vi "write key.vi"(8 "error in (no error)":errorcluster, 10 "key":u8, 11 "uri":string) -> (0 "error out":errorcluster, 2 "key out":u8, 3 "function return":i32)   [LabVIEW 2012, in "libximc.lvlib"]
doc: "result_t XIMC_API write_key (const char* uri, uint8_t* key);"
uses:
  libximc.lvlib
  libximc.dll
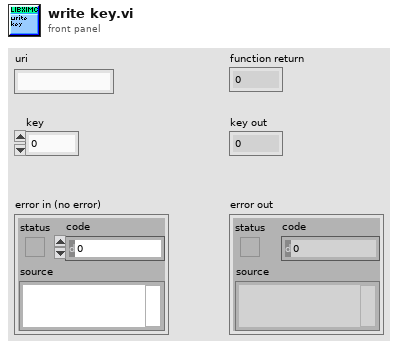
[diagram p1: front panel]
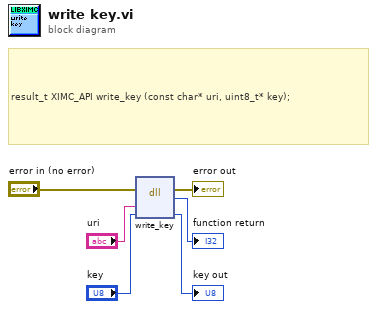
[diagram p0: block diagram]
diagram:
  # "result_t XIMC_API write_key (const char* uri, uint8_t* key);"
  n1 = dll-call lib="C:/Users/Vasily/Att_examples/LabVIEW_example/libximc.*" fn="write_key"(error in="error in (no error)", "uri"="uri", "key"="key") -> (error out=→"error out":errorcluster, →"function return":i32, "key"=→"key out":u8)  [unwired: 3 in, 1 out]
